vi "20211029_HW02.vi"() -> ()   [LabVIEW 2019]
panel:
  in  "Listbox":i32(listbox)=2
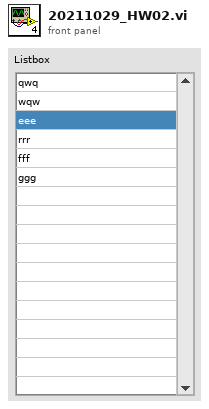
[diagram p1: front panel]
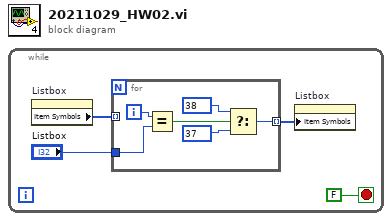
[diagram p0: block diagram]
diagram:
  n1 = while {
    stop <- FALSE stop-if-true
    n2 = property on="Listbox" class="LstBox (strict)"() -> ("Item Symbols"=w4:i32[])  [unwired: 2 in, 2 out]
    n3 = for {
      tunnel: w4 -> [_] mode=indexing
      tunnel: "Listbox" -> [w10]
      tunnel: [w6] -> w2 mode=indexing
      i -> [w5]
      n4 = Equal?(x=w5, y=w10) -> (x = y?=w9:bool)
      n5 = Select(t=38, s=w9, f=37) -> (s? t:f=w6:i32)
    }
    n6 = property on="Listbox" class="LstBox (strict)"("Item Symbols"=w2) -> ()  [unwired: 2 in, 2 out]
  }
